vi "Plotter_data.vi"(0 "Vari Spaced":dbl[][](array[numeric]) format="%.2f", 1 "Plot No":i32, 2 "Voltages":dbl[][](array[numeric]) format="%.2f", 5 "Equi Spaced":dbl[][](array[numeric]) format="%.2f", 7 "Histogram":dbl[][](array[numeric]) format="%.2f", 9 "Spectra":dbl[][](array[numeric]) format="%.2f", 11 "Auto-correlation":dbl[][](array[numeric]) format="%.2f", 12 "Graph":T2={"Plot 1"=1, "Plot 2"=3, "Save graph"=0, "Plot Type"=enum."Voltage trace"} {"Save graph" items=["Do not save plot", "Save plot"]; "Plot 2" items=["Nothing", "Velocity1", "Arr time1", "Velocity2", "Arr time2"]; "Plot 1" items=["Nothing", "Velocity1", "Arr time1", "Velocity2", "Arr time2"]}) -> (8 "Plot data":cluster{"Xo":dbl, "Delta X":dbl, dbl[]}[](array[cluster]) {"?" format="%.2f"; "Delta X" format="%.2f"; "Xo" format="%.2f"})   [LabVIEW 2010]
uses:
  Controls/Graph_Type.ctl
  Globals/Meas_global.vi
  Globals/LDA_meas_global_1.vi
  Acquisition/PWA/PWAtasksGLOBAL.vi
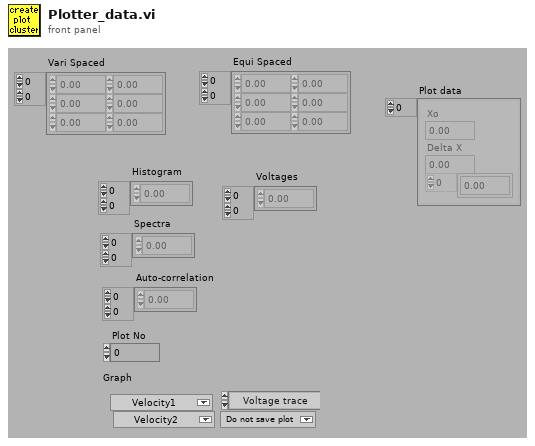
[diagram p1: front panel]
types:
  T1 = typedef "Graph_Type.ctl" = enum16{"Show no graph", "Voltage trace", "Velocity trace", "Vel histogram", "Spectrum", "f.E(f) v Log f", "Auto-Corr"}
  T2 = cluster{"Plot 1":u16, "Plot 2":u16, "Save graph":u16, "Plot Type":T1}
  T3 = cluster{"Insts for plotting[0]":u16, "Insts for plotting[1]":u16}
  T4 = typedef "Analysis_info_cluster.ctl" = cluster{"Colour":u32, "Inst type":T5, "Inst name":string, "Symbol":string, "Code name":string, "Extra Info":string, "Inst Array":T6, "Index":i32, "Voltage Index":i32, "Extra Titles":string[], "Extra Values":string[]}
  T5 = typedef "Inst_type.ctl" = enum16{"Propeller anemometer", "Raw voltage", "Pressure Transducer", "Pitot-static tube", "Preston tube", "Hot wire", "Cross wire 1", "Cross wire 2", "Generic Linear", "Generic Polynomial", "Generic BackPoly", "Fast FID", "Thermocouple", "Cold wire", "Pulsed Wire", "LDA Vel", "LDA Tran time", "LDA Arr time"}
  T6 = typedef "Instrument_Array.ctl" = enum16{"PWA", "LDA", "Analogue"}
  T7 = cluster{"Xo":dbl, "Delta X":dbl, "Auto-correlation":dbl[]}
  T8 = cluster{"Xo":dbl, "Delta X":dbl, "Auto-correlation":dbl[]}[]
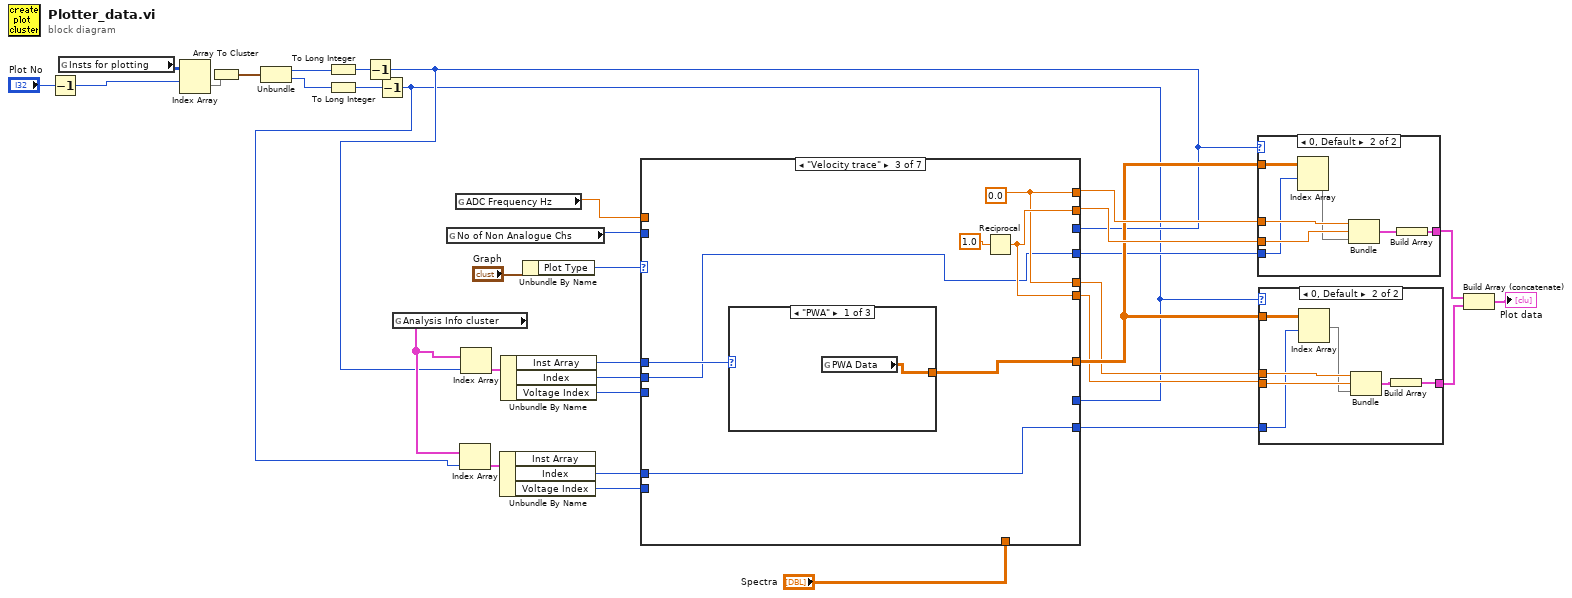
[diagram p0: block diagram]
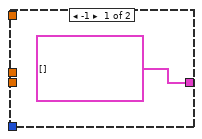
[diagram p2: hidden frame]
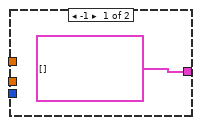
[diagram p3: hidden frame]
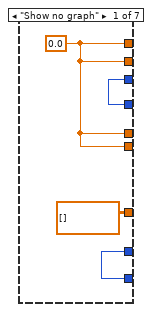
[diagram p4: hidden frame]
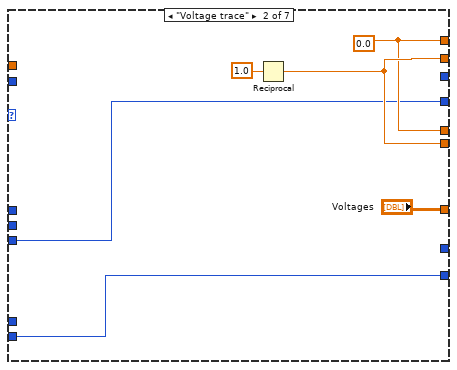
[diagram p5: hidden frame]
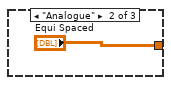
[diagram p6: hidden frame]
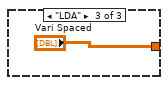
[diagram p7: hidden frame]
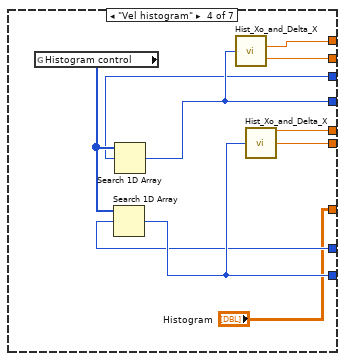
[diagram p8: hidden frame]
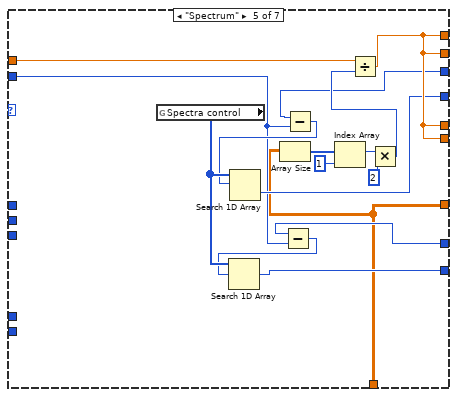
[diagram p9: hidden frame]
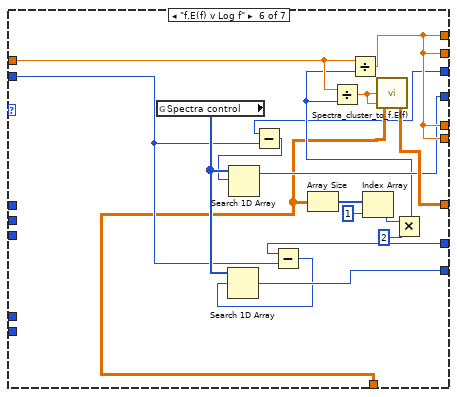
[diagram p10: hidden frame]
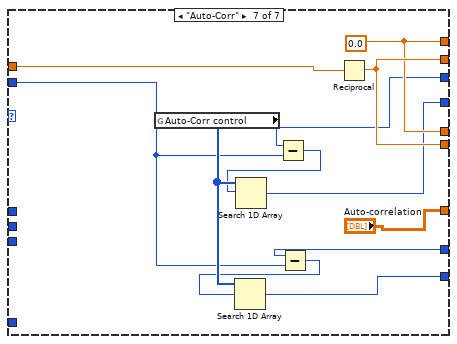
[diagram p11: hidden frame]
diagram:
  n1 = Decrement(x="Plot No") -> (x-1=w21:i32)
  n2 = global read "Meas_global.vi" "Insts for plotting"() -> (w27:u16[][])
  n3 = Index Array(array=w27, index (row)=w21) -> (element=w26:u16[])  [unwired: 1 in]
  n4 = Array To Cluster(array=w26) -> (cluster=w18:T3)
  n5 = Unbundle(w18) -> ("Insts for plotting[0]"=w17:u16, "Insts for plotting[1]"=w16:u16)
  n6 = To Long Integer(number=w17) -> (32bit integer=w14:i32)
  n7 = To Long Integer(number=w16) -> (32bit integer=w15:i32)
  n8 = Decrement(x=w14) -> (x-1=w3:i32)
  n9 = Decrement(x=w15) -> (x-1=w2:i32)
  n10 = global read "Meas_global.vi" "Analysis Info cluster"() -> (w9:T4[])
  n11 = global read "Meas_global.vi" "No of Non Analogue Chs"() -> (w12:i32)
  n12 = global read "LDA_meas_global_1.vi" "ADC Frequency Hz"() -> (w13:dbl)
  n13 = Index Array(array=w9, index=w2) -> (element=w10:T4)
  n14 = Index Array(array=w9, index=w3) -> (element=w11:T4)
  n15 = Unbundle By Name(w10) -> ("Index"=w4:i32, "Voltage Index"=w7:i32)  [unwired: 1 out]
  n16 = Unbundle By Name(w11) -> ("Inst Array"=w6:T6, "Index"=w5:i32, "Voltage Index"=w8:i32)
  n17 = Unbundle By Name("Graph") -> ("Plot Type"=w23:T1)
  n18 = case shown="\"Velocity trace\"" w23 {
    tunnel: [w38 w43 w50 w64 w79 w98 w108] -> w34
    tunnel: [w38 w44 w51 w63 w79 w98 w109] -> w33
    tunnel: [w38 w43 w50 w62 w79 w98 w108] -> w31
    tunnel: [w38 w44 w51 w61 w79 w98 w109] -> w30
    tunnel: w13 -> [_ _ _ _ w80 w96 w110]
    tunnel: [dbl[][] [] "Voltages" w47 "Histogram" w65 w95 "Auto-correlation"] -> w32
    tunnel: [w36 w40 w46 w59 w77 w93 w106] -> w20
    tunnel: [w35 w39 w45 w58 w76 w92 w105] -> w19
    tunnel: w12 -> [_ _ _ _ w72 w85 w104]
    tunnel: w8 -> [_ w40 _ _ _ _ _]
    tunnel: w7 -> [_ w39 _ _ _ _ _]
    tunnel: w6 -> [_ _ w48 _ _ _ _]
    tunnel: w5 -> [_ _ w46 _ _ _ _]
    tunnel: w4 -> [_ _ w45 _ _ _ _]
    tunnel: w3 -> [w36 _ _ w57 w66 w82 w99]
    tunnel: w2 -> [w35 _ _ w56 w67 w81 w100]
    tunnel: "Spectra" -> [_ _ _ _ w65 w83 _]
    frame "Show no graph" {
      w38 = 0.0
    }
    frame "Voltage trace" {
      w43 = 0.0
      n19 = Reciprocal(x=1.0) -> (1/x=w44:dbl)
    }
    frame "Velocity trace" {
      w50 = 0.0
      n20 = case shown="\"PWA\"" w48 {
        tunnel: [w52 "Equi Spaced" "Vari Spaced"] -> w47
        frame "PWA" {
          n21 = global read "PWAtasksGLOBAL.vi" "PWA Data"() -> (w52:dbl[][])
        }
        frame "Analogue" {
        }
        frame "LDA" {
        }
      }
      n22 = Reciprocal(x=1.0) -> (1/x=w51:dbl)
    }
    frame "Vel histogram" {
      n23 = global read "Meas_global.vi" "Histogram control"() -> (w60:i32[])
      n24 = Search 1D Array(1D array=w60, element=w56) -> (index of element=w58:i32)  [unwired: 1 out]
      n25 = Search 1D Array(1D array=w60, element=w57) -> (index of element=w59:i32)  [unwired: 1 out]
      n26 = call "Hist_Xo_and_Delta_X.vi"("Histogram index"=w59) -> ("Xo"=w64:dbl, "Delta X"=w63:dbl)  [unwired: 5 out]
      n27 = call "Hist_Xo_and_Delta_X.vi"("Histogram index"=w58) -> ("Xo"=w62:dbl, "Delta X"=w61:dbl)  [unwired: 5 out]
    }
    frame "Spectrum" {
      n28 = global read "Meas_global.vi" "Spectra control"() -> (w78:i32[])
      n29 = Array Size(array=w65) -> (size(s)=w74:i32[])
      n30 = Subtract(x=w67, y=w72) -> (x-y=w71:i32)
      n31 = Search 1D Array(1D array=w78, element=w71) -> (index of element=w76:i32)  [unwired: 1 out]
      n32 = Subtract(x=w66, y=w72) -> (x-y=w73:i32)
      n33 = Search 1D Array(1D array=w78, element=w73) -> (index of element=w77:i32)  [unwired: 1 out]
      n34 = Index Array(array=w74, index=1) -> (element=w70:i32)
      n35 = Multiply(x=w70, y=2) -> (x*y=w68:i32)
      n36 = Divide(x=w80, y=w68) -> (x/y=w79:dbl)
    }
    frame "f.E(f) v Log f" {
      n37 = global read "Meas_global.vi" "Spectra control"() -> (w94:i32[])
      n38 = Subtract(x=w82, y=w85) -> (x-y=w89:i32)
      n39 = Search 1D Array(1D array=w94, element=w89) -> (index of element=w93:i32)  [unwired: 1 out]
      n40 = Subtract(x=w81, y=w85) -> (x-y=w84:i32)
      n41 = Search 1D Array(1D array=w94, element=w84) -> (index of element=w92:i32)  [unwired: 1 out]
      n42 = Array Size(array=w83) -> (size(s)=w90:i32[])
      n43 = Index Array(array=w90, index=1) -> (element=w87:i32)
      n44 = Multiply(x=w87, y=2) -> (x*y=w86:i32)
      n45 = Divide(x=w96, y=w86) -> (x/y=w97:dbl)
      n46 = Divide(x=w96, y=w86) -> (x/y=w98:dbl)
      n47 = call "Spectra_cluster_to_f.E(f).vi"("delta f"=w97, "f"=w97, "Spectra array"=w83) -> ("f.E(f) array"=w95:dbl[][])
    }
    frame "Auto-Corr" {
      w108 = 0.0
      n48 = global read "Meas_global.vi" "Auto-Corr control"() -> (w107:i32[])
      n49 = Subtract(x=w99, y=w104) -> (x-y=w103:i32)
      n50 = Search 1D Array(1D array=w107, element=w103) -> (index of element=w106:i32)  [unwired: 1 out]
      n51 = Subtract(x=w100, y=w104) -> (x-y=w102:i32)
      n52 = Search 1D Array(1D array=w107, element=w102) -> (index of element=w105:i32)  [unwired: 1 out]
      n53 = Reciprocal(x=w110) -> (1/x=w109:dbl)
    }
  }
  n54 = case shown="0, Default" w3 {
    tunnel: w32 -> [_ w118]
    tunnel: w34 -> [_ w117]
    tunnel: w33 -> [_ w116]
    tunnel: [cluster{"Xo":dbl, "Delta X":dbl, dbl[]}[] [] w113] -> w29
    tunnel: w20 -> [_ w112]
    frame -1 {
    }
    frame 0, Default {
      n55 = Index Array(array=w118, index (row)=w112) -> (element=w115:dbl[])  [unwired: 1 in]
      n56 = Bundle("Xo"=w117, "Delta X"=w116, "Auto-correlation"=w115) -> (w114:T7)  [unwired: 1 out]
      n57 = Build Array(w114) -> (w113:T8)
    }
  }
  n58 = case shown="0, Default" w2 {
    tunnel: w32 -> [_ w126]
    tunnel: w31 -> [_ w125]
    tunnel: w30 -> [_ w124]
    tunnel: [cluster{"Xo":dbl, "Delta X":dbl, dbl[]}[] [] w121] -> w28
    tunnel: w19 -> [_ w120]
    frame -1 {
    }
    frame 0, Default {
      n59 = Index Array(array=w126, index (row)=w120) -> (element=w123:dbl[])  [unwired: 1 in]
      n60 = Bundle("Xo"=w125, "Delta X"=w124, "Auto-correlation"=w123) -> (w122:T7)  [unwired: 1 out]
      n61 = Build Array(w122) -> (w121:T8)
    }
  }
  n62 = Build Array (concatenate)(w29, w28) -> (→"Plot data":T8)
